vi "solar_qtimer Set Delay.vi"(6 "Suppress Errors? (T)":bool=TRUE, 7 "Target Name":string, 8 "error in (no error)":errorcluster, 9 "Delay (-1)":i32=-1, 10 "QTimer Name":string, 11 "QTimer Refnum in":T1) -> (0 "error out":errorcluster, 3 "QTimer Refnum out":T1)   [LabVIEW 2018]
doc: "This sets the delay of the QTimer by name."
uses:
  solar_qtimer_ctl Refnum.ctl
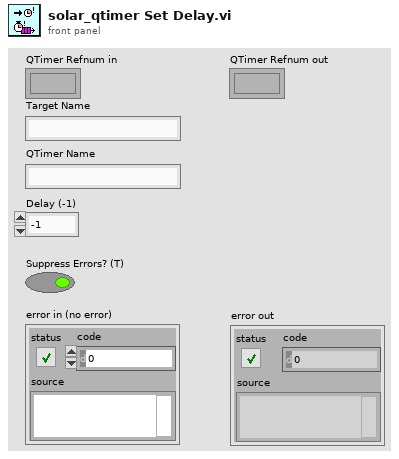
[diagram p1: front panel]
types:
  T1 = typedef "solar_qtimer_ctl Refnum.ctl" = refnum<k1>
  T2 = typedef "solar_qtimer_ctl SEQ.ctl" = cluster{"QTimers":T3[]}
  T3 = typedef "solar_qtimer_ctl QTimer.ctl" = cluster{"Settings":T4, "Queue":refnum<queue>, "QTimerQ":refnum<queue>, "VI Refnum":refnum<vi>}
  T4 = typedef "solar_qtimer_ctl QTimer Settings.ctl" = cluster{"QTimer":string, "Delay":i32, "Start":bool, "EnQ_Type":enum8{"Normal", "Priority", "IgnoreIfExists"}, "Messages":cluster{"MSG":string, "DATA":variant}[]}
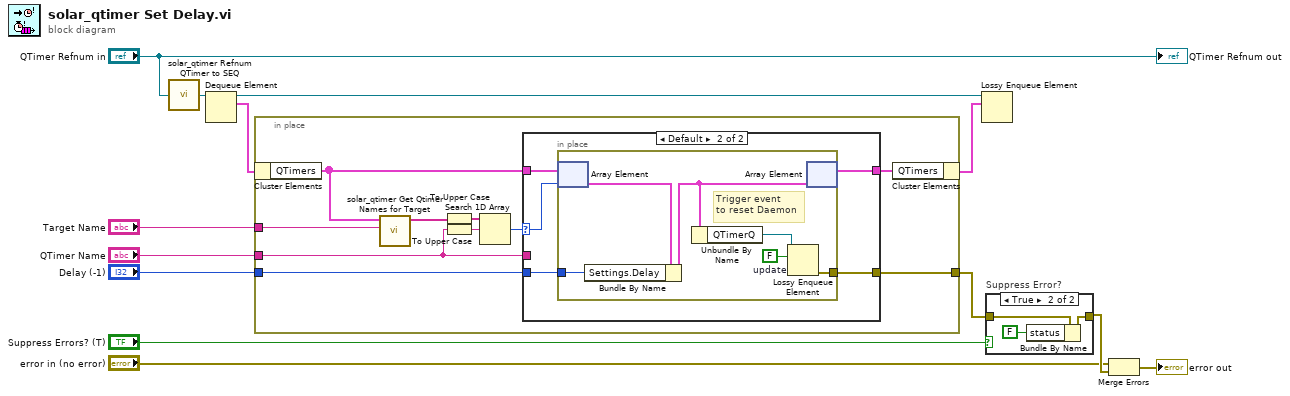
[diagram p0: block diagram]
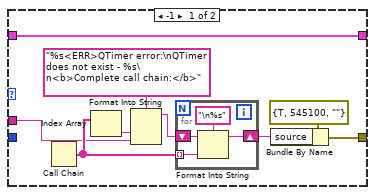
[diagram p2: hidden frame]
diagram:
  n1 = call "solar_qtimer Refnum QTimer to SEQ.vi"("QTimer Refnum"="QTimer Refnum in") -> ("QTimers SEQ"=w12:refnum<queue>)
  n2 = Dequeue Element(queue=w12) -> (queue out=w11:refnum<queue>, element=w10:T2)  [unwired: 2 in, 2 out]
  n3 = in-place {
    in-place-border: "QTimer Name" -> [w19]
    in-place-border: [w18] -> w5
    in-place-border: "Delay (-1)" -> [w17]
    in-place-border: "Target Name" -> [w14]
    n4 = in-place-cluster #1(w10) -> ("QTimers"=w15:T3[])
    n5 = call "solar_qtimer Get Qtimer Names for Target.vi"("Target Name"=w14, "QTimers"=w15) -> ("Target's Qtimer Names"=w16:string[])  [unwired: 9 in]
    n6 = To Upper Case(1:w16) -> (0:w23:string[])
    n7 = To Upper Case(1:w19) -> (0:w22:string)
    n8 = Search 1D Array(1D array=w23, element=w22) -> (index of element=w21:i32)  [unwired: 1 in]
    n9 = case shown="Default" w21 {
      selector: w21 -> [_ w40]
      tunnel: w15 -> [w32 w41]
      tunnel: [w32 w39] -> w20
      tunnel: w19 -> [w25 _]
      tunnel: [w24 w37] -> w18
      tunnel: w17 -> [_ w38]
      frame -1 {
        n10 = Call Chain() -> (call chain=w28:string[])
        n11 = Index Array(array=w28) -> (element=w30:string)  [unwired: 1 in]
        n12 = Format Into String(format string="%s<ERR>QTimer error:\nQTimer does not exist - %s\n<b>Complete call chain:</b>", w30, w25) -> (resulting string=w29:string)  [unwired: 2 in, 1 out]
        n13 = for {
          tunnel: w28 -> [w36] mode=indexing
          shift-right: [w35] -> w27
          shift-left: w29 -> [w34]
          n14 = Format Into String(format string="\n%s", initial string=w34, w36) -> (resulting string=w35:string)  [unwired: 1 in, 1 out]
        }
        n15 = Bundle By Name(cluster=errorcluster {"status"=TRUE, "code"=545100, "source"=""} ("error in (no error)"), "source"=w27) -> (w24:errorcluster)
      }
      frame Default {
        n16 = in-place {
          in-place-border: w38 -> [w46]
          in-place-border: [w44] -> w37
          w43 = FALSE  # update
          # "Trigger event\nto reset Daemon"
          n17 = in-place-array #2(w41, w40) -> (w47:T3)
          n18 = Bundle By Name(cluster=w47, "Settings.Delay"=w46) -> (w45:T3)
          n19 = Unbundle By Name(w45) -> ("QTimerQ"=w42:refnum<queue>)
          n20 = Lossy Enqueue Element(queue=w42, element=w43) -> (error out=w44:errorcluster)  [unwired: 1 in, 3 out]
          n21 = in-place-array #2(w45) -> (w39:T3[])  [unwired: 1 out]
        }
      }
    }
    n22 = in-place-cluster #1("QTimers"=w20) -> (w9:T2)
  }
  n23 = Lossy Enqueue Element(queue=w11, element=w9) -> ()  [unwired: 1 in, 4 out]
  n24 = case "Suppress Error?" shown="True" "Suppress Errors? (T)" {
    tunnel: w5 -> [w48 w51]
    tunnel: [w48 w50] -> w6
    frame False {
    }
    frame True {
      n25 = Bundle By Name(cluster=w51, "status"=FALSE) -> (w50:errorcluster)
    }
  }
  n26 = Merge Errors("error in (no error)", w6) -> (→"error out":errorcluster)
  "QTimer Refnum out" <- "QTimer Refnum in"
